vi "initialize timing source.vi"(8 "error in":errorcluster, 11 "timing source in":refnum<class "scan engine timing source.lvclass">) -> (0 "error out":errorcluster, 3 "timing source out":refnum<class "scan engine timing source.lvclass">)   [LabVIEW 2013, in "scan engine timing source.lvclass"]
doc: "An interface for initializing a timing source. In many cases this may be a no-op. There is no expectation about when this function should be called, but it must be called before entering the loop to be timed."
uses:
  scan engine timing source.lvclass
  scan engine timing source.lvclass/scan engine timing source.ctl
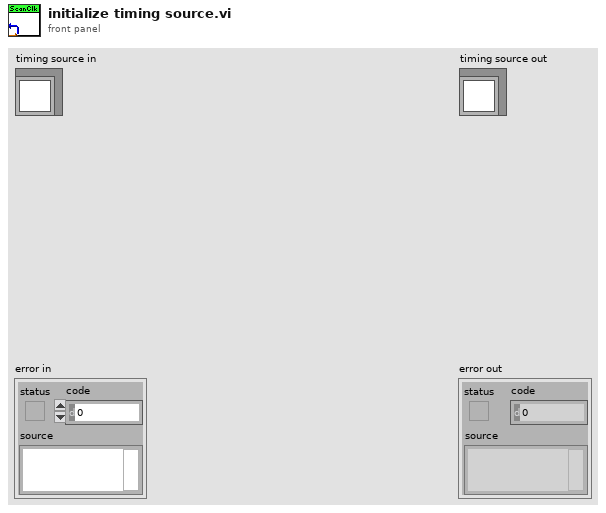
[diagram p1: front panel]
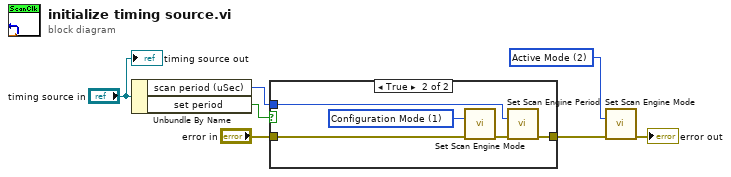
[diagram p0: block diagram]
diagram:
  w3 = 2 items=["Configuration Mode"=1, "Active Mode"=2] ("mode (Active Mode)")
  n1 = Unbundle By Name("timing source in") -> ("scan period (uSec)"=w5:u32, "set period"=w4:bool)
  n2 = case shown="True" w4 {
    tunnel: [w8 w9] -> w2
    tunnel: "error in" -> [w8 w11]
    tunnel: w5 -> [_ w10]
    frame False {
    }
    frame True {
      w12 = 1 items=["Configuration Mode"=1, "Active Mode"=2] ("mode (Active Mode)")
      n3 = call <vilib>:"Set Scan Engine Mode.vi"("mode (Active Mode)"=w12, "error in (no error)"=w11) -> ("error out"=w13:errorcluster)  [unwired: 13 in]
      n4 = call <vilib>:"Set Scan Engine Period.vi"("scan period (uSec)"=w10, "error in (no error)"=w13) -> ("error out"=w9:errorcluster)  [unwired: 13 in]
    }
  }
  n5 = call <vilib>:"Set Scan Engine Mode.vi"("mode (Active Mode)"=w3, "error in (no error)"=w2) -> ("error out"=→"error out":errorcluster)  [unwired: 13 in]
  "timing source out" <- "timing source in"
